vi "updateSpec.vi"(9 "profile":waveform(dbl), 11 "spectrum":waveform(dbl)) -> (5 "time:updateSpec":u32)   [LabVIEW 2013, in "MagAnalysis_Online.lvclass"]
uses:
  MagAnalysis_Online.lvclass
  shared/CompressAndUpdate(Poly)/CompressAndUpdate(String).vi
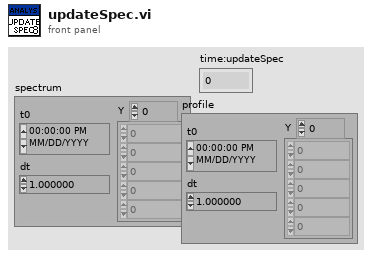
[diagram p1: front panel]
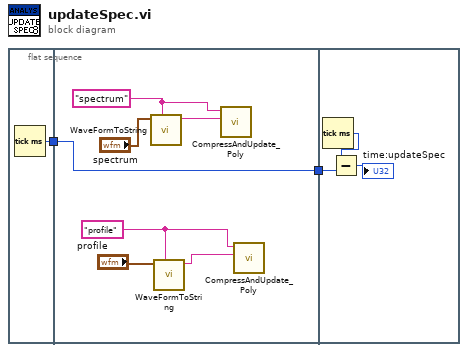
[diagram p0: block diagram]
diagram:
  n1 = flat-sequence {
    tunnel: [w3] -> w2
    tunnel: w2 -> [w8]
    tunnel: [w8] -> w1
    tunnel: w1 -> [w12]
    frame #0 {
      n2 = Tick Count (ms)() -> (millisecond timer value=w3:u32)
    }
    frame #1 {
      w4 = "profile" ("channelName")
      w6 = "spectrum" ("channelName")
      n3 = call "WaveFormToString.vi"("channelName"=w6, "Waveform"="spectrum") -> ("string"=w9:string)  [unwired: 9 in]
      n4 = call "WaveFormToString.vi"("channelName"=w4, "Waveform"="profile") -> ("string"=w5:string)  [unwired: 9 in]
      n5 = call-poly "CompressAndUpdate_Poly.vi"("String"=w9, "command or variable name"=w6) -> ()  [unwired: 9 in, 1 out]
      n6 = call-poly "CompressAndUpdate_Poly.vi"("String"=w5, "command or variable name"=w4) -> ()  [unwired: 9 in, 1 out]
    }
    frame #2 {
      n7 = Tick Count (ms)() -> (millisecond timer value=w13:u32)
      n8 = Subtract(x=w13, y=w12) -> (x-y=→"time:updateSpec":u32)
    }
  }
